vi "LockinDAQ.GetPublicEvents.vi"(8 "error in (no error)":errorcluster, 11 "LockinDAQ":refnum<class "LockinDAQ.lvclass">) -> (0 "error out":errorcluster, 2 "LIADAQ Public Events":T1, 3 "LockinDAQ out":refnum<class "LockinDAQ.lvclass">)   [LabVIEW 2016, in "LockinDAQ.lvclass"]
doc: "---------------------------------------------------------------\nJKI State Machine Objects™\nhttp://jki.net/state-machine-objects/\nCopyright (C) 2005-2015, JKI <info@jki.net>\nALL RIGHTS RESERVEDJKI State Machine Objects (SMO) 1.0.0.4\nJKI - JKI\nCopyright (c) 2015, JKI"
uses:
  LockinDAQ.lvclass
  Typedefs/PublicEvents--Cluster.ctl
  Typedefs/PublicEvents--LockinDAQ.getAO.ctl
  Typedefs/PublicEvents--LockinDAQ.getAI.ctl
  Typedefs/PublicEvents--LockinDAQ.getREF.ctl
  Typedefs/PublicEvents--LockinDAQ.getResults.ctl
  Typedefs/Results--Cluster.ctl
  Typedefs/PublicEvents--LockinDAQ.getCalibration.ctl
  Typedefs/PublicEvents--LockinDAQ.getAOChannels.ctl
  Typedefs/AO-cluster.ctl
  Typedefs/Function-enum.ctl
  Typedefs/PublicEvents--LockinDAQ.getREFChannels.ctl
  Typedefs/REF-cluster.ctl
  Typedefs/PublicEvents--LockinDAQ.getDAQState.ctl
  Typedefs/State-enum.ctl
  Typedefs/PublicEvents--LockinDAQ.getSweepResults.ctl
  Typedefs/SweepResults--Cluster.ctl
  LockinDAQ.lvclass/LockinDAQ.ctl
panel:
  # "For instructions on how to use the JKI State Machine Objects, examples and video tutorials, visit:\nhttp://jki.net/state-machine-objects/\n\nJKI State Machine Objects™\nhttp://jki.net/state-machine-objects/\nCopyright (C) 2005-2015, JKI <info@jki.net>\nALL RIGHTS RESERVED"
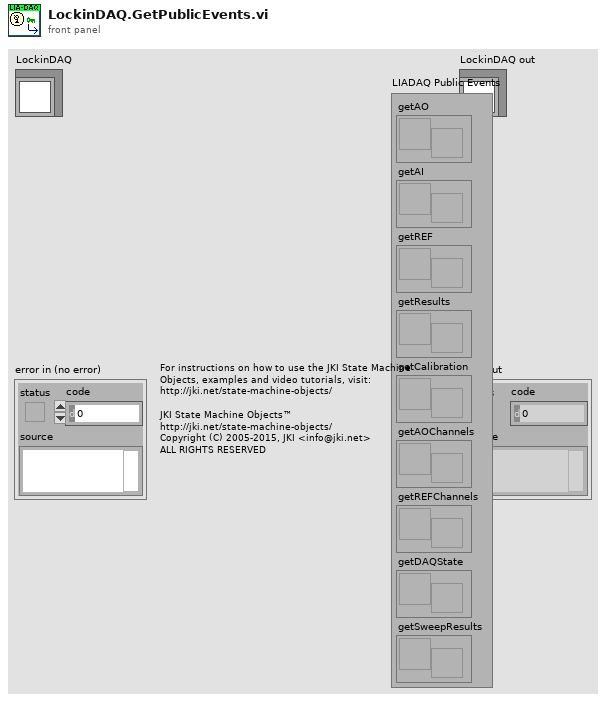
[diagram p1: front panel]
types:
  T1 = typedef "LockinDAQ.lvclass/PublicEvents--Cluster.ctl" = cluster{"getAO":refnum<user-event>, "getAI":refnum<user-event>, "getREF":refnum<user-event>, "getResults":refnum<user-event>, "getCalibration":refnum<user-event>, "getAOChannels":refnum<user-event>, "getREFChannels":refnum<user-event>, "getDAQState":refnum<user-event>, "getSweepResults":refnum<user-event>}
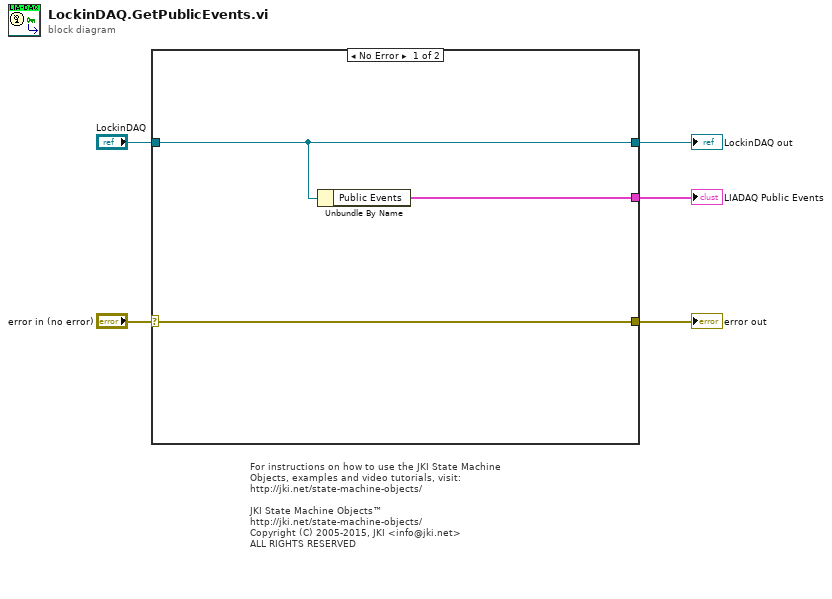
[diagram p0: block diagram]
diagram:
  # "For instructions on how to use the JKI State Machine Objects, examples and video tutorials, visit:\nhttp://jki.net/state-machine-objects/\n\nJKI State Machine Objects™\nhttp://jki.net/state-machine-objects/\nCopyright (C) 2005-2015, JKI <info@jki.net>\nALL RIGHTS RESERVED"
  n1 = case shown="No Error" "error in (no error)" {
    selector: "error in (no error)" -> [w7 w9]
    tunnel: "LockinDAQ" -> [w6 w10]
    tunnel: [w7 w9] -> w4
    tunnel: [w6 w10] -> w3
    tunnel: [w8 _] -> w1
    frame No Error {
      n2 = Unbundle By Name(w6) -> ("Public Events"=w8:T1)
    }
    frame Error {
    }
  }
  "error out" <- w4
  "LockinDAQ out" <- w3
  "LIADAQ Public Events" <- w1
